vi "PhotometricElectricTestingAutomation - Main.vi"() -> ()   [LabVIEW 2013]
doc: "Use this template to build a standard state machine design pattern. Each state executes code and determines which state to transition to. Contrast this design pattern with the User Interface Event Handler pattern, in which code executes in response to user actions. Contrast this design pattern also with the Queued Message Handler pattern, in which each message handling code can queue zero or more new messages.\nNote: This template does not contain the most recent programming guidelines recommended by National Instruments. For a complete, project-based implementation of the Standard State Machine pattern, use the Create Project dialog box instead of this template."
uses:
  Functions/Electrical Measurements/Controls/electrical.ctl
  Functions/Electrical Measurements/Controls/StateMachineStates.ctl
  Libraries/California Instruments iX Series/California Instruments iX Series.lvlib
panel:
  in  "Tab Control":T1(tab)
  in  "Voltage Level (0V)":dbl=120.0
  out "Next State":T2
  out "Electrical Data":T3
  in  "Turn On Source":bool
  in  "Electrical Refnum in":refnum<visa-resource-name>
  out "error out":errorcluster
  in  "error in (no error)":errorcluster
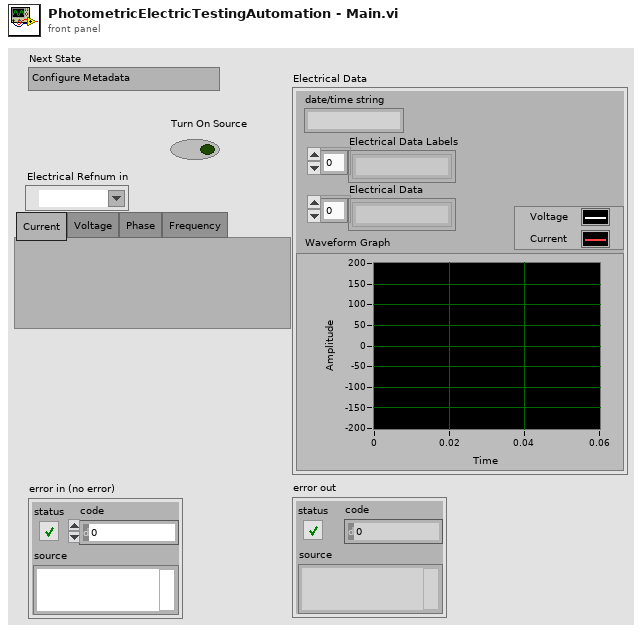
[diagram p1: front panel]
types:
  T1 = enum32{"Current", "Voltage", "Phase", "Frequency"}
  T2 = typedef "StateMachineStates.ctl" = enum16{"Configure Metadata", "Initialize", "Idle", "Calibration", "Aux Correction", "Stabilize", "Take Measurement", "Check If Data is Good", "Notify Operator", "Stop"}
  T3 = typedef "electrical.ctl" = cluster{"date/time string":string, "Electrical Data Labels":string[], "Electrical Data":string[], "Waveform Graph":waveform(dbl)[]}
  T4 = cluster{string, "Electrical data labels":string[], string[], "Waveform Graph":waveform(sgl)[]}
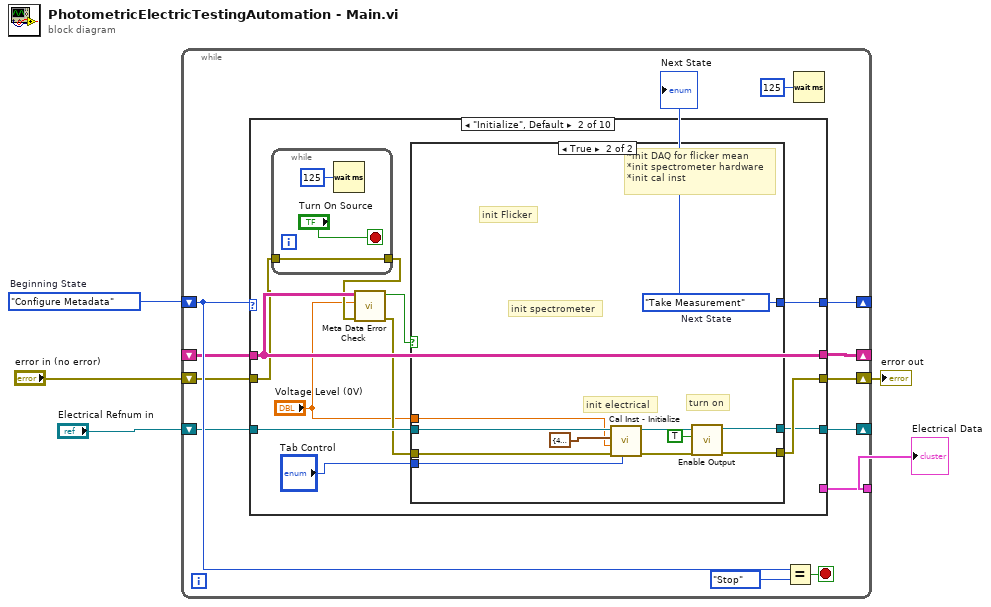
[diagram p0: block diagram]
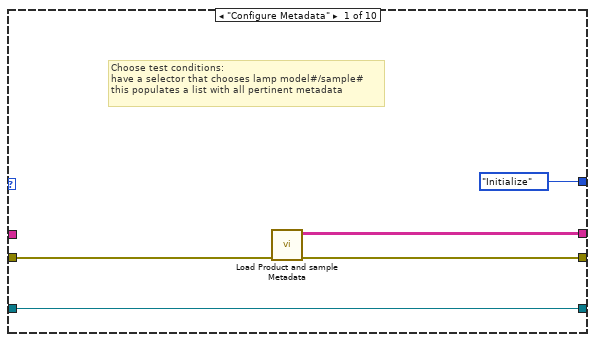
[diagram p2: hidden frame]
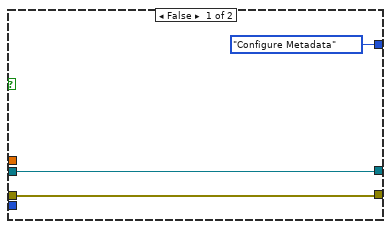
[diagram p3: hidden frame]
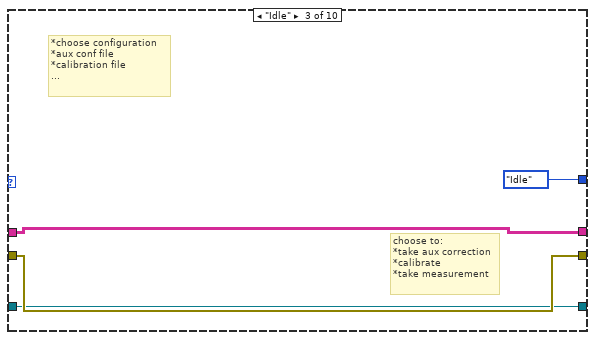
[diagram p4: hidden frame]
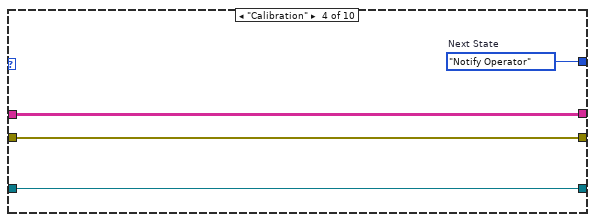
[diagram p5: hidden frame]
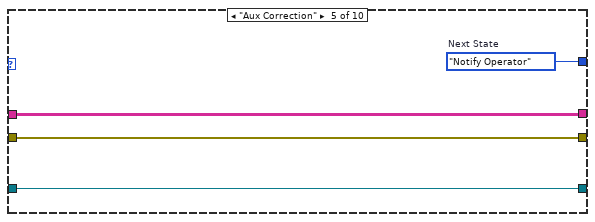
[diagram p6: hidden frame]
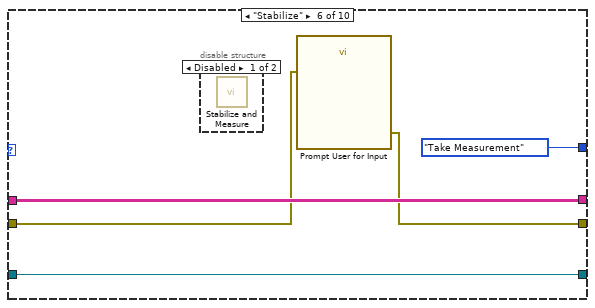
[diagram p7: hidden frame]
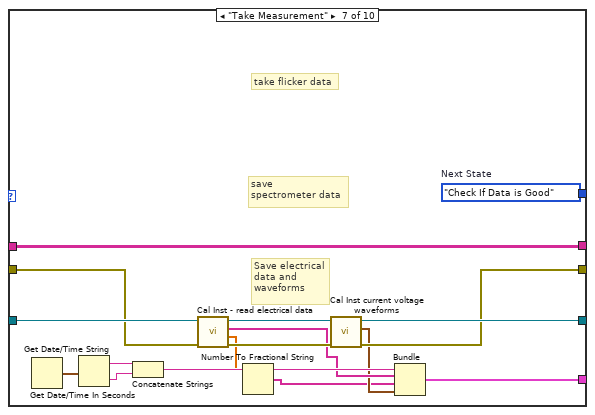
[diagram p9: hidden frame]
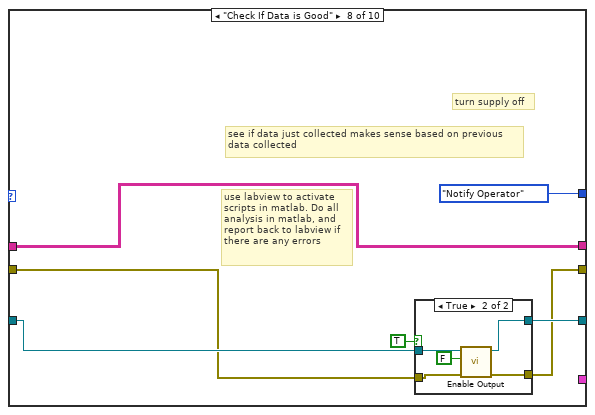
[diagram p10: hidden frame]
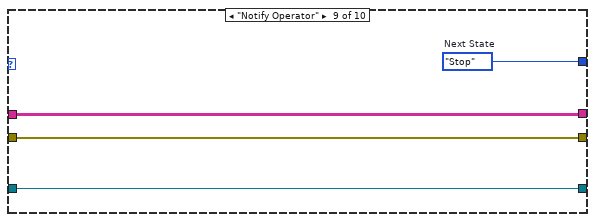
[diagram p12: hidden frame]
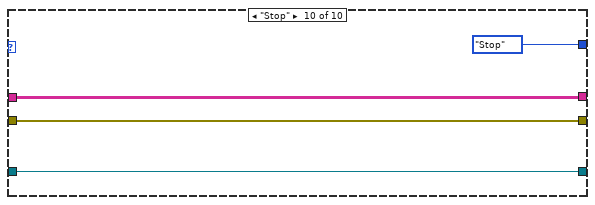
[diagram p13: hidden frame]
diagram:
  w5 = StateMachineStates."Configure Metadata"  # Beginning State
  n1 = while {
    shift-right: [w14] -> _
    shift-left: w5 -> [w15]
    shift-right: [w11] -> _
    shift-left: _ -> [w10]
    shift-right: [w12] -> w4
    shift-left: "error in (no error)" -> [w9]
    shift-right: [w8] -> _
    shift-left: "Electrical Refnum in" -> [w7]
    tunnel: [w6] -> w1
    stop <- w17 stop-if-true
    n2 = case shown="\"Initialize\", Default" w15 {
      tunnel: [StateMachineStates."Initialize" ("Next State") w33 StateMachineStates."Idle" ("Next State") w58 w62 StateMachineStates."Take Measurement" ("Next State") w84 StateMachineStates."Notify Operator" ("Next State") w102 StateMachineStates."Stop" ("Next State")] -> w14
      tunnel: [w21 w31 w52 w56 w60 w63 w77 w85 w100 w104] -> w12
      tunnel: [w20 w29 w53 w57 w61 w67 w83 w90 w101 w105] -> w11
      tunnel: w10 -> [_ w29 w53 w57 w61 w67 w83 w90 w101 w105]
      tunnel: w9 -> [w19 w26 w52 w56 w60 w64 w78 w86 w100 w104]
      tunnel: [w18 w30 w51 w55 w59 w66 w80 w88 w99 w103] -> w8
      tunnel: w7 -> [w18 w32 w51 w55 w59 w66 w82 w89 w99 w103]
      tunnel: [_ _ _ _ _ _ w70 _ _ _] -> w6
      frame "Configure Metadata" {
        # "Choose test conditions:\nhave a selector that chooses lamp model#/sample#\nthis populates a list with all pertinent metadata"
        n3 = call "Load Product and sample Metadata.vi"("error in (no error)"=w19) -> ("error out"=w21:errorcluster, "Meta Data"=w20:string[][])  [unwired: 9 in]
      }
      frame "Initialize", Default {
        n4 = while {
          tunnel: w26 -> [w35]
          tunnel: [w35] -> w25
          stop <- "Turn On Source" stop-if-true
          n5 = Wait (ms)(milliseconds to wait=u32 125) -> ()  [unwired: 1 out]
        }
        n6 = call "Meta Data Error Check.vi"("error in (no error)"=w25, "Voltage Level (0V)"="Voltage Level (0V)", "Meta Data"=w29) -> ("error out"=w28:errorcluster, "No Error"=w27:bool)  [unwired: 7 in]
        n7 = case shown="True" w27 {
          tunnel: [StateMachineStates."Configure Metadata" ("Next State") w50] -> w33
          tunnel: w28 -> [w39 w48]
          tunnel: w32 -> [w38 w47]
          tunnel: [w39 w44] -> w31
          tunnel: [w38 w43] -> w30
          tunnel: "Tab Control" -> [_ w41]
          tunnel: "Voltage Level (0V)" -> [_ w40]
          frame False {
          }
          frame True {
            w50 = StateMachineStates."Take Measurement"  # Next State
            # "turn on"
            # "init electrical"
            # "init spectrometer"
            # "init Flicker"
            # "*init DAQ for flicker mean\n*init spectrometer hardware\n*init cal inst"
            n8 = call "Cal Inst - Initialize.vi"("Tab Control"=w41, "error in (no error)"=w48, "Voltage Level (0V)"=w40, "Serial Configuration"=cluster{"Baud Rate":u32, "Flow Control":u16} {"Baud Rate"=460800, "Flow Control"=0}, "VISA Refnum in"=w47) -> ("error out"=w45:errorcluster, "VISA Refnum out"=w46:refnum<visa-resource-name>)  [unwired: 5 in]
            n9 = call "Enable Output.vi"("error in (no error)"=w45, "Enable Output (T: Enable)"=TRUE, "VISA resource name"=w46) -> ("error out"=w44:errorcluster, "VISA resource name out"=w43:refnum<visa-resource-name>)  [unwired: 7 in]
          }
        }
      }
      frame "Idle" {
        # "choose to:\n*take aux correction\n*calibrate\n*take measurement"
        # "*choose configuration\n*aux conf file\n*calibration file\n..."
      }
      frame "Calibration" {
        w58 = StateMachineStates."Notify Operator"  # Next State
      }
      frame "Aux Correction" {
        w62 = StateMachineStates."Notify Operator"  # Next State
      }
      frame "Stabilize" {
        n10 = disable-structure shown="Disabled" {
          frame Disabled {
            n11 = call "Stabilize and Measure.vi"() -> ()  [unwired: 11 in, 1 out]
          }
          frame Enabled {
          }
        }
        n12 = call "Prompt User for Input"("error in (no error)"=w64) -> ("error out"=w63:errorcluster)  [unwired: 17 in, 1 out]
      }
      frame "Take Measurement" {
        w84 = StateMachineStates."Check If Data is Good"  # Next State
        # "take flicker data"
        # "save\nspectrometer data"
        # "Save electrical\ndata and\nwaveforms"
        n13 = Get Date/Time In Seconds() -> (seconds since 1Jan1904=w76:timestamp)
        n14 = Get Date/Time String(seconds (now)=w76) -> (date string=w75:string, time string=w74:string)  [unwired: 2 in]
        n15 = Concatenate Strings(w75, w74) -> (w73:string)
        n16 = call "Cal Inst - read electrical data.vi"("error in (no error)"=w78, "VISA Refnum in"=w82) -> ("error out"=w79:errorcluster, "Electrical Data"=w69:dbl[], "Electrical data labels"=w72:string[], "VISA Refnum out"=w81:refnum<visa-resource-name>)  [unwired: 6 in]
        n17 = Number To Fractional String(number=w69) -> (F-format string=w68:string[])  [unwired: 3 in]
        n18 = call "Cal Inst current voltage waveforms.vi"("error in (no error)"=w79, "VISA resource name"=w81) -> ("error out"=w77:errorcluster, "Waveform Graph"=w71:waveform(sgl)[], "VISA resource name out"=w80:refnum<visa-resource-name>)  [unwired: 7 in]
        n19 = Bundle(w73, "Electrical data labels"=w72, w68, "Waveform Graph"=w71) -> (w70:T4)  [unwired: 1 in]
      }
      frame "Check If Data is Good" {
        # "turn supply off"
        # "use labview to activate\nscripts in matlab. Do all\nanalysis in matlab, and \nreport back to labview if\nthere are any errors"
        # "see if data just collected makes sense based on previous\ndata collected"
        n20 = case shown="True" TRUE {
          tunnel: w89 -> [w93 w98]
          tunnel: [w93 w97] -> w88
          tunnel: w86 -> [w92 w95]
          tunnel: [w92 w94] -> w85
          frame False {
          }
          frame True {
            n21 = call "Enable Output.vi"("error in (no error)"=w95, "Enable Output (T: Enable)"=FALSE, "VISA resource name"=w98) -> ("error out"=w94:errorcluster, "VISA resource name out"=w97:refnum<visa-resource-name>)  [unwired: 7 in]
          }
        }
      }
      frame "Notify Operator" {
        w102 = StateMachineStates."Stop"  # Next State
      }
      frame "Stop" {
      }
    }
    "Next State" <- w14
    n22 = Equal?(x=w15, y=StateMachineStates."Stop" ("States")) -> (x = y?=w17:bool)
    n23 = Wait (ms)(milliseconds to wait=u32 125) -> ()  [unwired: 1 out]
  }
  "error out" <- w4
  "Electrical Data" <- w1
